vi "Update and Increase Velocity.vi"(8 "Increase":dbl, 9 "Hit Lower Boundary?":bool, 10 "Hit Upper Boundary?":bool, 11 "Velocity":dbl) -> (3 "Updated Velocity":dbl)   [LabVIEW 2015]
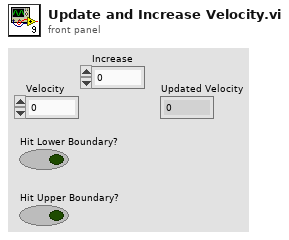
[diagram p1: front panel]
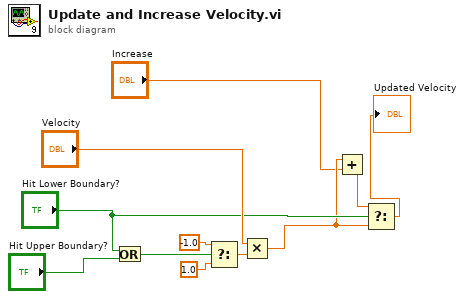
[diagram p0: block diagram]
diagram:
  n1 = Or(x="Hit Lower Boundary?", y="Hit Upper Boundary?") -> (x .or. y?=w11:bool)
  n2 = Select(t=-1.0, s=w11, f=1.0) -> (s? t:f=w6:dbl)
  n3 = Multiply(x="Velocity", y=w6) -> (x*y=w4:dbl)
  n4 = Add(x=w4, y="Increase") -> (x+y=w3:dbl)
  n5 = Select(t=w3, s="Hit Lower Boundary?", f=w4) -> (s? t:f=→"Updated Velocity":dbl)
